vi "Wysyllanie danych do PC .vi"(5 "remote port":u16, 6 "odczytany CAN":T1 {"type" items=["CAN Data", "CAN Remote"]; "identifier" format="%.0x"}, 7 "Numeric":u32, 8 "error in (no error)":errorcluster, 11 "UDP Network Connection in":refnum<k16>) -> (0 "error out":errorcluster, 3 "UDP Network Connection out":refnum<k16>)   [LabVIEW 2015]
uses:
  <vilib>/RioEmbeddedCAN/RioEmbeddedCAN.llb/CANFrameControl.ctl
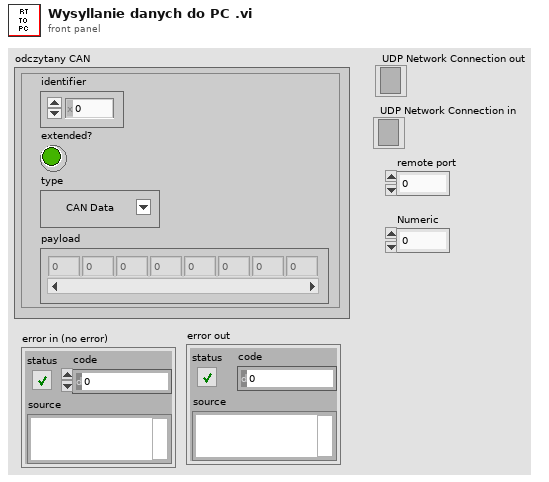
[diagram p1: front panel]
types:
  T1 = typedef "CANFrameControl.ctl" = cluster{"identifier":u32, "extended?":bool, "type":u8, "payload":u8[]}
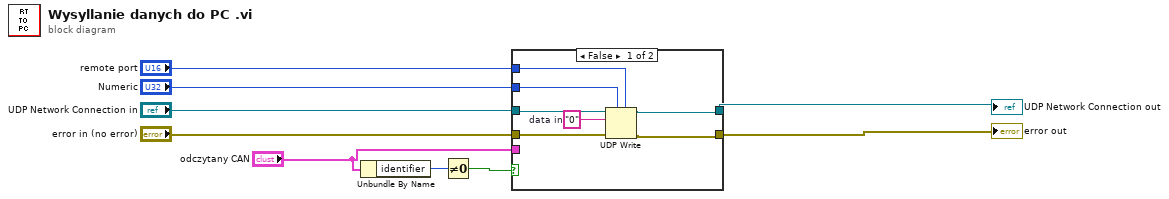
[diagram p0: block diagram]
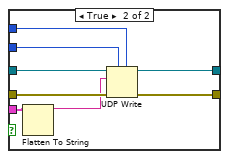
[diagram p2: hidden frame]
diagram:
  n1 = Unbundle By Name("odczytany CAN") -> ("identifier"=w1:u32)
  n2 = Not Equal To 0?(x=w1) -> (x != 0?=w4:bool)
  n3 = case shown="False" w4 {
    tunnel: [w14 w24] -> w8
    tunnel: "Numeric" -> [w11 w23]
    tunnel: "remote port" -> [w10 w22]
    tunnel: "UDP Network Connection in" -> [w16 w21]
    tunnel: "error in (no error)" -> [w15 w20]
    tunnel: [w13 w19] -> w9
    tunnel: "odczytany CAN" -> [_ w18]
    frame False {
      w12 = "0"  # data in
      n4 = UDP Write(address=w11, port or service name=w10, connection ID=w16, data in=w12, 8:w15) -> (error out=w13:errorcluster, 3:w14:refnum<k16>)  [unwired: 1 in]
    }
    frame True {
      n5 = Flatten To String(anything=w18) -> (data string=w17:string)  [unwired: 3 in, 2 out]
      n6 = UDP Write(address=w23, port or service name=w22, connection ID=w21, data in=w17, 8:w20) -> (error out=w19:errorcluster, 3:w24:refnum<k16>)  [unwired: 1 in]
    }
  }
  "error out" <- w9
  "UDP Network Connection out" <- w8
